vi "Manipulators_Control_Alg.vi"(9 "Op_1_Bumpers":bool, 10 "Op2_Buttons":T1, 11 "Op2_Joysticks":cluster{"Z":i32, "LeftY":i32, "RightY":i32} {"RightY" scale=-37626.0..37626.0; "LeftY" scale=-37626.0..37626.0; "Z" scale=-37626.0..37626.0}) -> (1 "SolenoidsOut":bool[](array[boolean]), 3 "MotorsOut":u16[](array[slide]) scale=0.0..512.0)   [LabVIEW 2013, in "ProcessorHelperFunctions.lvlib"]
uses:
  ProcessorHelperFunctions.lvlib
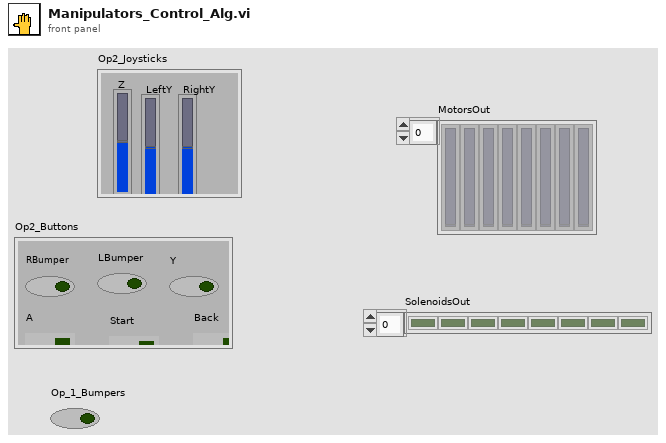
[diagram p1: front panel]
types:
  T1 = cluster{"RBumper":bool, "LBumper":bool, "Y":bool, "A":bool, "Start":bool, "Back":bool}
  T2 = cluster{"JoystickOut[0]":i32, "JoystickOut[1]":i32, "JoystickOut[2]":i32, "JoystickOut[3]":i32, "JoystickOut[4]":i32, "JoystickOut[5]":i32, "JoystickOut[6]":i32, "JoystickOut[7]":i32, "JoystickOut[8]":i32}
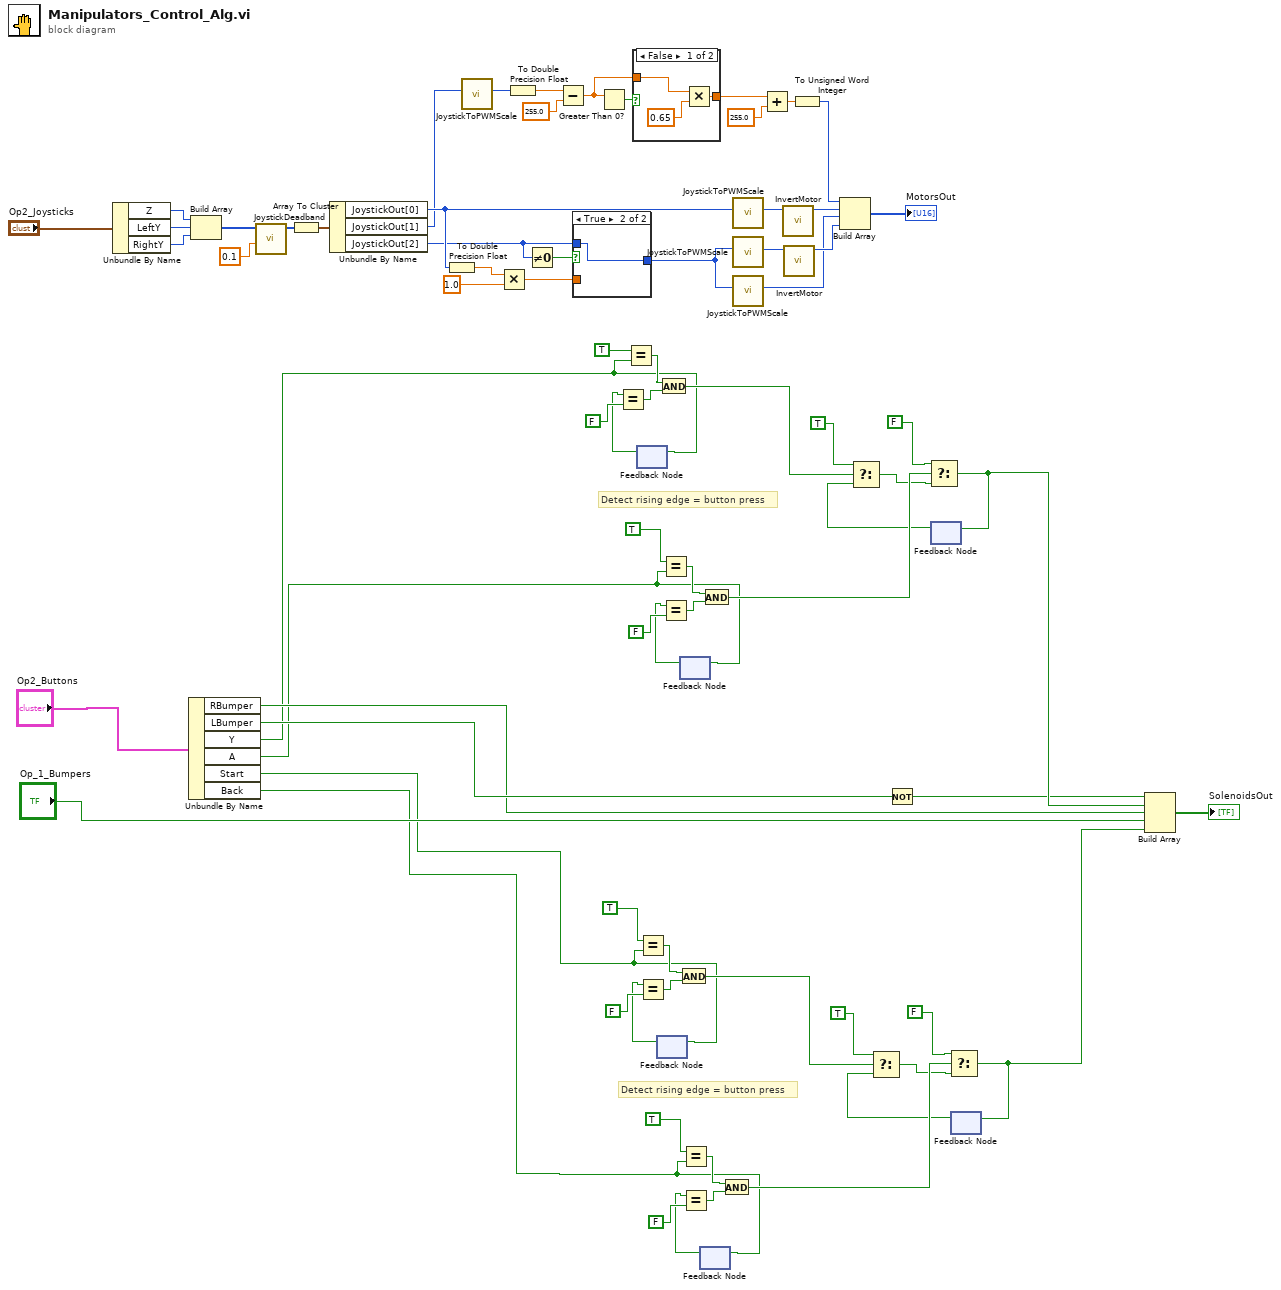
[diagram p0: block diagram]
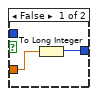
[diagram p2: hidden frame]
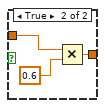
[diagram p3: hidden frame]
diagram:
  # "Detect rising edge = button press"
  # "Detect rising edge = button press"
  n1 = Unbundle By Name("Op2_Joysticks") -> ("Z"=w29:i32, "LeftY"=w28:i32, "RightY"=w27:i32)
  n2 = Unbundle By Name("Op2_Buttons") -> ("RBumper"=w70:bool, "LBumper"=w71:bool, "Y"=w52:bool, "A"=w51:bool, "Start"=w33:bool, "Back"=w32:bool)
  n3 = Build Array(w29, w28, w27) -> (w26:i32[])
  n4 = call "JoystickDeadband.vi"("DBPercent"=0.1, "JoystickIn"=w26) -> ("JoystickOut"=w24:i32[])  [unwired: 9 in]
  n5 = Array To Cluster(array=w24) -> (cluster=w23:T2)
  n6 = Unbundle By Name(w23) -> ("JoystickOut[0]"=w11:i32, "JoystickOut[1]"=w7:i32, "JoystickOut[2]"=w6:i32)
  n7 = To Double Precision Float(number=w11) -> (double precision float=w10:dbl)
  n8 = call "JoystickToPWMScale.vi"("Numeric"=w7) -> ("Numeric 2"=w15:u16)  [unwired: 10 in]
  n9 = Multiply(x=w10, y=1.0) -> (x*y=w5:dbl)
  n10 = To Double Precision Float(number=w15) -> (double precision float=w14:dbl)
  n11 = Not Equal To 0?(x=w6) -> (x != 0?=w8:bool)
  n12 = Subtract(x=w14, y=255.0) -> (x-y=w21:dbl)
  n13 = case shown="True" w8 {
    tunnel: w6 -> [_ w78]
    tunnel: w5 -> [w76 _]
    tunnel: [w77 w78] -> w4
    frame False {
      n14 = To Long Integer(number=w76) -> (32bit integer=w77:i32)
    }
    frame True {
    }
  }
  n15 = Greater Than 0?(x=w21) -> (x > 0?=w22:bool)
  n16 = Equal?(x=TRUE, y=w52) -> (x = y?=w64:bool)
  n17 = case shown="False" w22 {
    tunnel: w21 -> [w80 w84]
    tunnel: [w79 w82] -> w19
    frame False {
      n18 = Multiply(x=w80, y=0.65) -> (x*y=w79:dbl)
    }
    frame True {
      n19 = Multiply(x=w84, y=0.6) -> (x*y=w82:dbl)
    }
  }
  n20 = feedback #1() -> (w67:bool)  [unwired: 1 in]
  n21 = Equal?(x=w67, y=FALSE) -> (x = y?=w65:bool)
  n22 = feedback-in #1(w52) -> ()
  n23 = Equal?(x=TRUE, y=w33) -> (x = y?=w45:bool)
  n24 = feedback #2() -> (w48:bool)  [unwired: 1 in]
  n25 = Equal?(x=w48, y=FALSE) -> (x = y?=w46:bool)
  n26 = feedback-in #2(w33) -> ()
  n27 = And(x=w64, y=w65) -> (x .and. y?=w58:bool)
  n28 = Equal?(x=TRUE, y=w51) -> (x = y?=w59:bool)
  n29 = And(x=w45, y=w46) -> (x .and. y?=w39:bool)
  n30 = feedback #3() -> (w62:bool)  [unwired: 1 in]
  n31 = Equal?(x=w62, y=FALSE) -> (x = y?=w60:bool)
  n32 = feedback-in #3(w51) -> ()
  n33 = Equal?(x=TRUE, y=w32) -> (x = y?=w40:bool)
  n34 = feedback #4() -> (w43:bool)  [unwired: 1 in]
  n35 = Equal?(x=w43, y=FALSE) -> (x = y?=w41:bool)
  n36 = feedback-in #4(w32) -> ()
  n37 = And(x=w59, y=w60) -> (x .and. y?=w57:bool)
  n38 = And(x=w40, y=w41) -> (x .and. y?=w38:bool)
  n39 = call "JoystickToPWMScale.vi"("Numeric"=w11) -> ("Numeric 2"=w13:u16)  [unwired: 10 in]
  n40 = call "JoystickToPWMScale.vi"("Numeric"=w4) -> ("Numeric 2"=w3:u16)  [unwired: 10 in]
  n41 = call "JoystickToPWMScale.vi"("Numeric"=w4) -> ("Numeric 2"=w1:u16)  [unwired: 10 in]
  n42 = Add(x=w19, y=255.0) -> (x+y=w17:dbl)
  n43 = call "InvertMotor.vi"("Input"=w13) -> ("Output"=w12:u16)  [unwired: 10 in]
  n44 = call "InvertMotor.vi"("Input"=w3) -> ("Output"=w2:u16)  [unwired: 10 in]
  n45 = To Unsigned Word Integer(number=w17) -> (unsigned 16bit integer=w16:u16)
  n46 = Build Array(w16, w12, w1, w2) -> (→"MotorsOut":u16[])
  n47 = Not(x=w71) -> (.not. x?=w30:bool)
  n48 = feedback #5() -> (w54:bool)  [unwired: 1 in]
  n49 = Select(t=TRUE, s=w58, f=w54) -> (s? t:f=w56:bool)
  n50 = Select(t=FALSE, s=w57, f=w56) -> (s? t:f=w50:bool)
  n51 = feedback-in #5(w50) -> ()
  n52 = feedback #6() -> (w35:bool)  [unwired: 1 in]
  n53 = Select(t=TRUE, s=w39, f=w35) -> (s? t:f=w37:bool)
  n54 = Select(t=FALSE, s=w38, f=w37) -> (s? t:f=w31:bool)
  n55 = feedback-in #6(w31) -> ()
  n56 = Build Array(w30, w50, w70, "Op_1_Bumpers", w31) -> (→"SolenoidsOut":bool[])
